vi "HP81110A Query Patt Mem Data Into String.vi"(8 "error in (no error)":errorcluster, 10 "Channel (1:Channel 1)":T1(ring)=enum."Channel 1", 11 "VISA session":refnum<visa-resource-name>) -> (0 "error out":errorcluster, 1 "No Of Values":i32, 2 "output string":string, 3 "dup VISA session":refnum<visa-resource-name>)   [LabVIEW 2009]
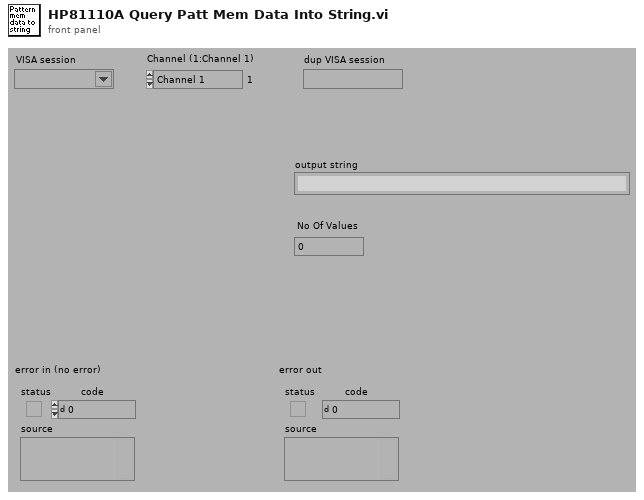
[diagram p1: front panel]
types:
  T1 = enum16{"Invalid", "Channel 1", "Channel 2", "Channel 3"}
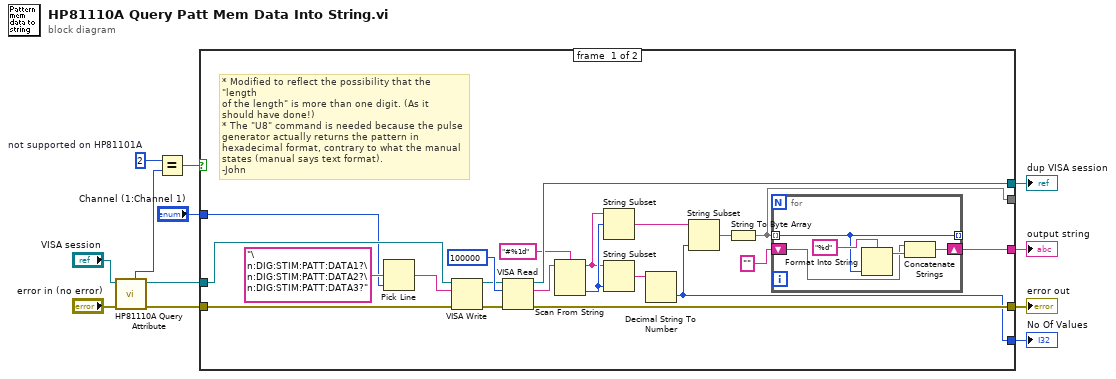
[diagram p0: block diagram]
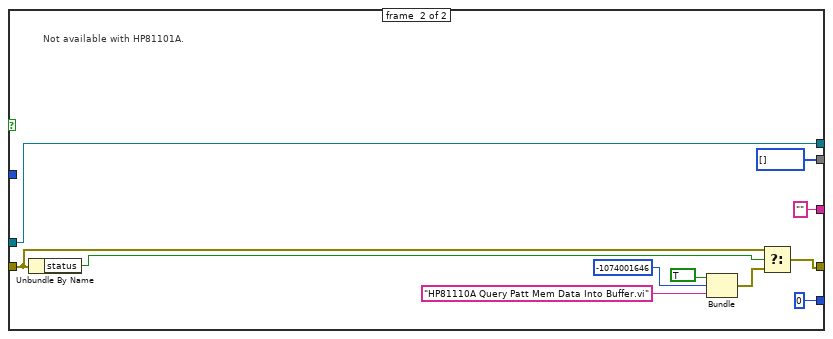
[diagram p2: hidden frame]
diagram:
  w8 = u32 2  # not supported on HP81101A
  n1 = call "HP81110A Query Attribute.vi"("error in (no error)"="error in (no error)", "VISA session"="VISA session") -> ("error out"=w6:errorcluster, "dup VISA session"=w5:refnum<visa-resource-name>, "Instr Version"=w9:u32)  [unwired: 7 out]
  n2 = Equal?(x=w8, y=w9) -> (x = y?=w3:bool)
  n3 = case shown="True" w3 {
    tunnel: w6 -> [w32 w44]
    tunnel: w5 -> [w31 w43]
    tunnel: [w18 0] -> w10
    tunnel: [w15 u8[] []] -> _
    tunnel: [w29 w43] -> w11
    tunnel: [w28 w42] -> w1
    tunnel: "Channel (1:Channel 1)" -> [w24 _]
    tunnel: [w13 ""] -> w2
    frame #0 {
      # "* Modified to reflect the possibility that the \"length \nof the length\" is more than one digit. (As it \nshould have done!)  \n* The \"U8\" command is needed because the pulse \ngenerator actually returns the pattern in \nhexadecimal format, contrary to what the manual\nstates (manual says text format).\n-John"
      n4 = Pick Line(multi-line string="\n:DIG:STIM:PATT:DATA1?\n:DIG:STIM:PATT:DATA2?\n:DIG:STIM:PATT:DATA3?", line index=w24) -> (output string=w33:string)  [unwired: 1 out]
      n5 = VISA Write(VISA resource name=w31, write buffer=w33, error in (no error)=w32) -> (VISA resource name out=w27:refnum<visa-resource-name>, error out=w26:errorcluster)  [unwired: 1 out]
      n6 = VISA Read(VISA resource name=w27, byte count=u32 100000 ("byte count (0)"), error in (no error)=w26) -> (VISA resource name out=w29:refnum<visa-resource-name>, read buffer=w17:string, error out=w28:errorcluster)  [unwired: 1 out]
      n7 = Scan From String(format string="#%1d", input string=w17) -> (remaining string=w21:string, output 1=w22:i32)  [unwired: 2 in, 3 out]
      n8 = String Subset(string=w21, offset (0)=w22) -> (substring=w19:string)  [unwired: 1 out]
      n9 = String Subset(string=w21, length (rest)=w22) -> (substring=w20:string)  [unwired: 1 out]
      n10 = Decimal String To Number(string=w20) -> (number=w18:i32)  [unwired: 3 out]
      n11 = String Subset(string=w19, length (rest)=w18) -> (substring=w16:string)  [unwired: 1 out]
      n12 = String To Byte Array(string=w16) -> (unsigned byte array=w15:u8[])
      n13 = for {
        tunnel: [w37] -> _ mode=indexing
        tunnel: w15 -> [w37] mode=indexing
        shift-right: [w35] -> w13
        shift-left: "" -> [w34]
        n14 = Format Into String(format string="%d", w37) -> (resulting string=w36:string)  [unwired: 2 in, 1 out]
        n15 = Concatenate Strings(w34, w36) -> (w35:string)
      }
    }
    frame #1 {
      # "Not available with HP81101A."
      n16 = Unbundle By Name(w44) -> ("status"=w49:bool)
      n17 = Bundle("status"=TRUE, "code"=-1074001646, "source"="HP81110A Query Patt Mem Data Into Buffer.vi") -> (w45:errorcluster)  [unwired: 1 out]
      n18 = Select(t=w44, s=w49, f=w45) -> (s? t:f=w42:errorcluster)
    }
  }
  "No Of Values" <- w10
  "error out" <- w1
  "dup VISA session" <- w11
  "output string" <- w2
